vi "RB2 parse the data.vi"(0 "Nav String":string="$,G,43,13,230,P,10,20,120,T,10,10,330,L,14,36,110,A,3,5,B,7,8,C,16,20,D,-1,-1,S,08,12,234\r", 1 "Jeep":string="G") -> (2 "Jeep Data":cluster{"Header":string, i32, i32}, 3 "Time":cluster{i32, i32, i32}, 4 "Valid?":bool)   [LabVIEW 2012]
doc: "This VI find the position of the tug, X, Y and Heading convered into grid values. The position values are positions on the occupancy grid, the heading is in degrees. It also finds the buoy locations in grid values and the time in hrs, min , secs."
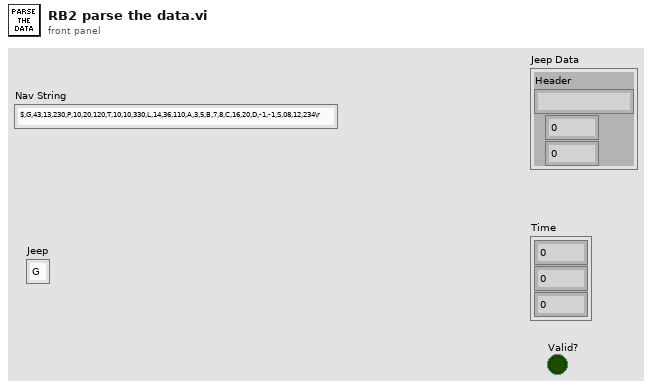
[diagram p1: front panel]
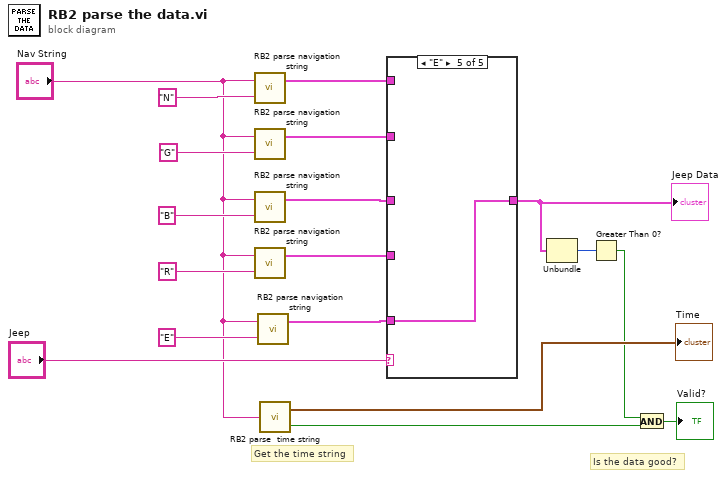
[diagram p0: block diagram]
diagram:
  # "Is the data good?"
  # "Get the time string"
  n1 = call "RB2 parse navigation string.vi"("Header"="N", "Nav String"="Nav String") -> ("Jeep Data"=w12:cluster{"Header":string, i32, i32})  [unwired: 1 out]
  n2 = call "RB2 parse navigation string.vi"("Header"="G", "Nav String"="Nav String") -> ("Jeep Data"=w11:cluster{"Header":string, i32, i32})  [unwired: 1 out]
  n3 = call "RB2 parse navigation string.vi"("Header"="B", "Nav String"="Nav String") -> ("Jeep Data"=w9:cluster{"Header":string, i32, i32})  [unwired: 1 out]
  n4 = call "RB2 parse navigation string.vi"("Header"="R", "Nav String"="Nav String") -> ("Jeep Data"=w8:cluster{"Header":string, i32, i32})  [unwired: 1 out]
  n5 = call "RB2 parse navigation string.vi"("Header"="E", "Nav String"="Nav String") -> ("Jeep Data"=w7:cluster{"Header":string, i32, i32})  [unwired: 1 out]
  n6 = call "RB2 parse  time string.vi"("Nav String"="Nav String") -> ("output cluster"=→"Time":cluster{i32, i32, i32}, "Valid?"=w3:bool)
  n7 = case shown="\"E\"" "Jeep" {
    tunnel: w12 -> [w19 _ _ _ _]
    tunnel: w11 -> [_ w20 _ _ _]
    tunnel: w9 -> [_ _ w21 _ _]
    tunnel: w8 -> [_ _ _ w22 _]
    tunnel: w7 -> [_ _ _ _ w23]
    tunnel: [w19 w20 w21 w22 w23] -> w6
    frame "N", Default {
    }
    frame "G" {
    }
    frame "B" {
    }
    frame "R" {
    }
    frame "E" {
    }
  }
  "Jeep Data" <- w6
  n8 = Unbundle(w6) -> (w5:i32)  [unwired: 2 out]
  n9 = Greater Than 0?(x=w5) -> (x > 0?=w2:bool)
  n10 = And(x=w2, y=w3) -> (x .and. y?=→"Valid?":bool)
